vi "Abort.vi"(8 "Error In":errorcluster, 11 "Keithley 6485 In":refnum<visa-resource-name>) -> (0 "Error Out":errorcluster, 3 "Keithley 6485 Out":refnum<visa-resource-name>)   [LabVIEW 2012, in "Keithley-6485.lvlib"]
uses:
  Keithley-6485.lvlib
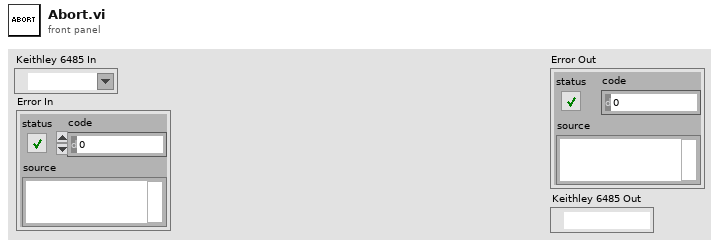
[diagram p1: front panel]
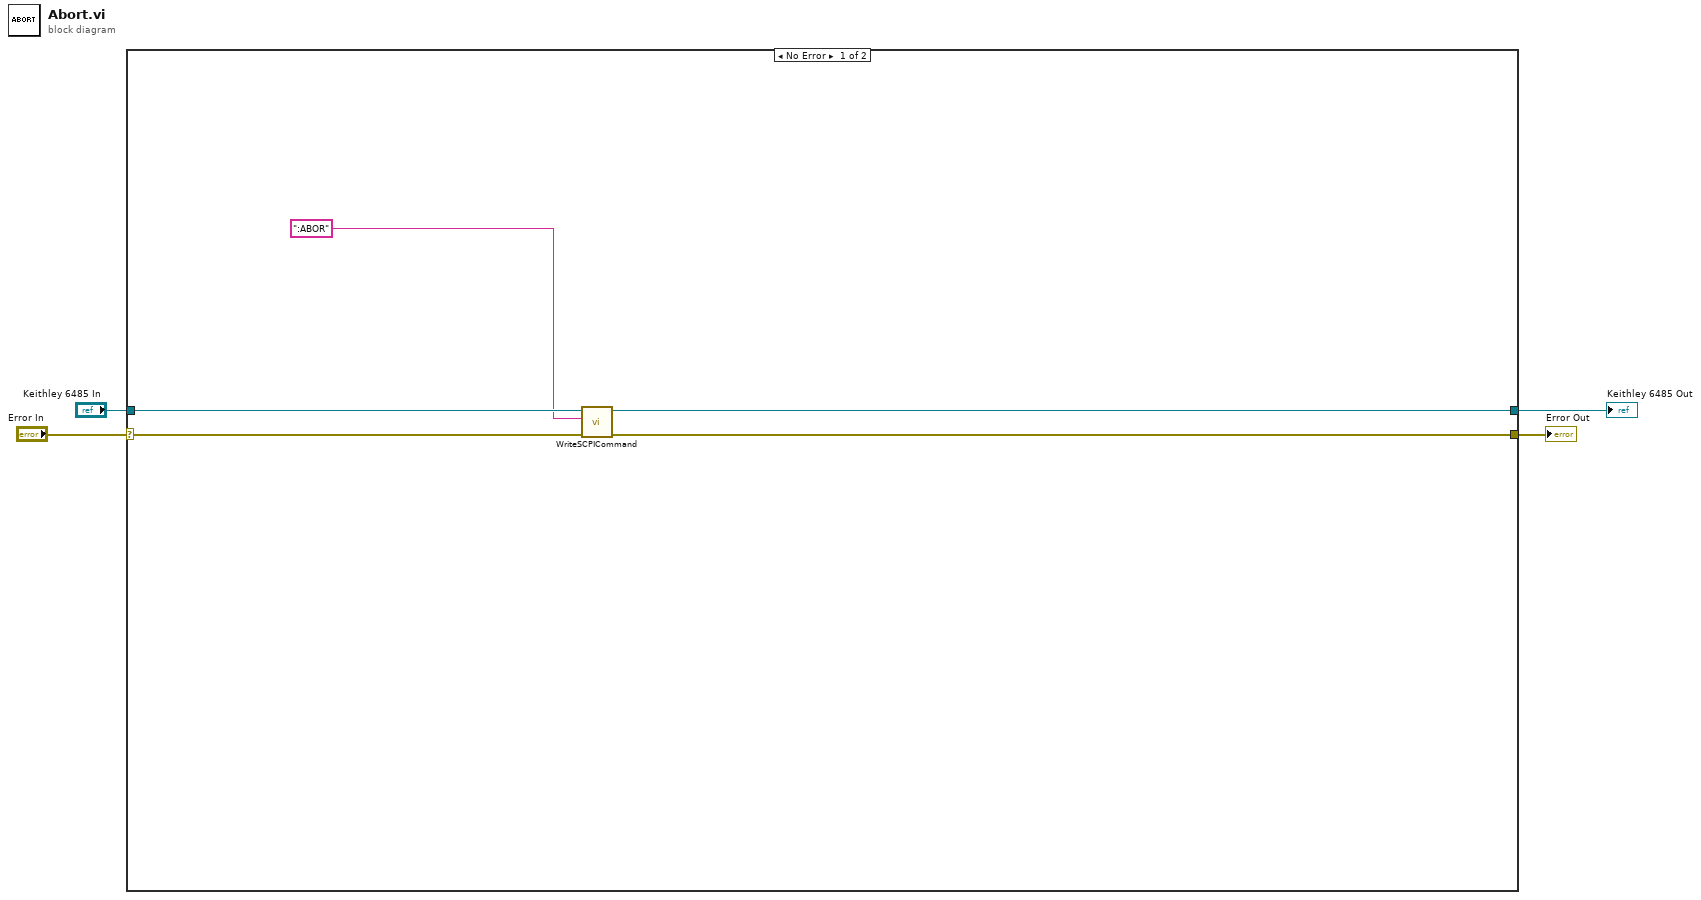
[diagram p0: block diagram]
diagram:
  n1 = case shown="No Error" "Error In" {
    selector: "Error In" -> [w9 w10]
    tunnel: "Keithley 6485 In" -> [w8 w11]
    tunnel: [w6 w10] -> w2
    tunnel: [w7 w11] -> w1
    frame No Error {
      n2 = call "WriteSCPICommand.vi"("Error In"=w9, "SCPI Command"=":ABOR" ("string"), "Keithley 6482 In"=w8) -> ("Error Out"=w6:errorcluster, "Keithley 6482 Out"=w7:refnum<visa-resource-name>)  [unwired: 7 in]
    }
    frame Error {
    }
  }
  "Error Out" <- w2
  "Keithley 6485 Out" <- w1
